vi "check Resource Array-PPS.vi"(8 "error in":errorcluster, 11 "Resource names":string[](array[string])) -> (0 "error out":errorcluster, 1 "Slave resource names":string[](array[string]), 2 "Single/Master resouce names":string, 3 "Single or ganged configuration":bool)   [LabVIEW 2021]
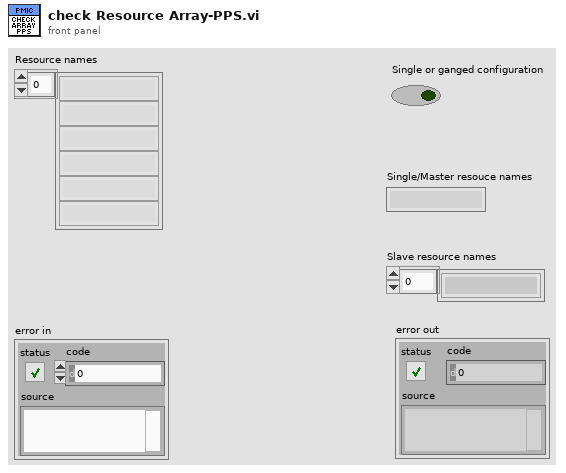
[diagram p1: front panel]
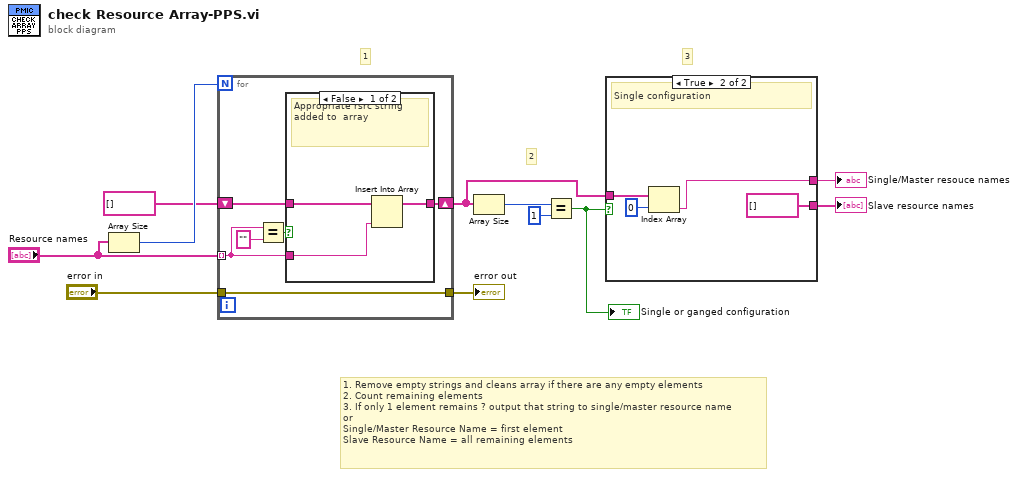
[diagram p0: block diagram]
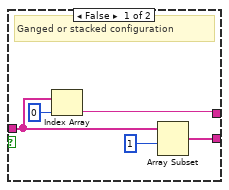
[diagram p2: hidden frame]
diagram:
  # "3"
  # "2"
  # "1"
  # "1. Remove empty strings and cleans array if there are any empty elements\n2. Count remaining elements\n3. If only 1 element remains ? output that string to single/master resource name \nor\nSingle/Master Resource Name = first element\nSlave Resource Name = all remaining elements"
  n1 = Array Size(array="Resource names") -> (size(s)=w11:i32)
  n2 = for {
    N: w11 -> [_]
    tunnel: "Resource names" -> [w13] mode=indexing
    shift-right: [w12] -> w1
    shift-left: string[] [] -> [w17]
    tunnel: "error in" -> [w16]
    tunnel: [w16] -> w8
    n3 = Equal?(x=w13, y="") -> (x = y?=w14:bool)
    n4 = case shown="False" w14 {
      tunnel: w17 -> [w20 w21]
      tunnel: w13 -> [w19 _]
      tunnel: [w18 w21] -> w12
      frame False {
        # "Appropriate rsrc string added to  array"
        n5 = Insert Into Array(array=w20, new element=w19) -> (w18:string[])  [unwired: 1 in]
      }
      frame True {
        # "Empty rsrc string removal from array"
      }
    }
  }
  "error out" <- w8
  n6 = Array Size(array=w1) -> (size(s)=w5:i32)
  n7 = Equal?(x=w5, y=1) -> (x = y?=w3:bool)
  "Single or ganged configuration" <- w3
  n8 = case shown="True" w3 {
    tunnel: w1 -> [w22 w30]
    tunnel: [w25 w28] -> w7
    tunnel: [w23 string[] []] -> w6
    frame False {
      # "Ganged or stacked configuration"
      n9 = Index Array(array=w22, index=0) -> (element=w25:string)
      n10 = Array Subset(array=w22, index=1) -> (w23:string[])  [unwired: 1 in]
    }
    frame True {
      # "Single configuration"
      n11 = Index Array(array=w30, index=0) -> (element=w28:string)
    }
  }
  "Single/Master resouce names" <- w7
  "Slave resource names" <- w6
